vi "Create Transfer Configuration.vi"(7 "base transfer name (transfer)":string="transfer", 11 "channel count per transfer":i32) -> (3 "transfer configuration":T1)   [LabVIEW 2017]
uses:
  DSF.Shared.Refactor.Typedefs.Transfer Configuration.ctl
  DSF.Shared.Typedefs.Byte Order.ctl
  DSF.Shared.Refactor.Typedefs.Channel Array Configuration.ctl
  DSF.Shared.Typedefs.Data Type.ctl
  DSF.Shared.lvlib
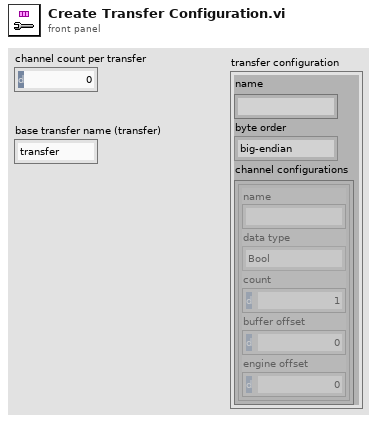
[diagram p1: front panel]
types:
  T1 = typedef "DSF.Shared.lvlib/DSF.Shared.Refactor.Typedefs.Transfer Configuration.ctl" = cluster{"name":string, "byte order":T2, "channel configurations":T3[]}
  T2 = typedef "DSF.Shared.lvlib/DSF.Shared.Typedefs.Byte Order.ctl" = enum8{"big-endian", "little-endian"}
  T3 = typedef "DSF.Shared.lvlib/DSF.Shared.Refactor.Typedefs.Channel Array Configuration.ctl" = cluster{"name":string, "data type":T4, "count":u64, "buffer offset":u64, "engine offset":u64}
  T4 = typedef "DSF.Shared.lvlib/DSF.Shared.Typedefs.Data Type.ctl" = enum8{"Bool", "SGL", "DBL", "I8", "I16", "I32", "I64", "U8", "U16", "U32", "U64"}
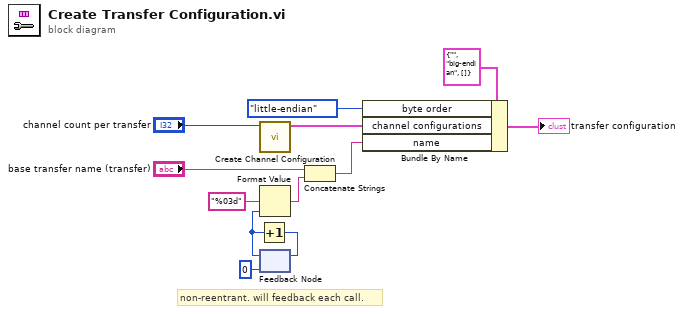
[diagram p0: block diagram]
diagram:
  # "non-reentrant. will feedback each call."
  n1 = call "Create Channel Configuration.vi"("channel count"="channel count per transfer") -> ("channel configurations"=w2:T3[])  [unwired: 9 in, 1 out]
  n2 = feedback #1(0) -> (w8:i32)
  n3 = Increment(x=w8) -> (x+1=w9:i32)
  n4 = Format Value(format string="%03d", value (0)=w8) -> (output string=w3:string)  [unwired: 1 in]
  n5 = feedback-in #1(w9) -> ()
  n6 = Concatenate Strings("base transfer name (transfer)", w3) -> (w1:string)
  n7 = Bundle By Name(cluster=T1 {"name"="", "byte order"=enum."big-endian", "channel configurations"=[]} ("Transfer Configuration"), "byte order"=DSF.Shared.Typedefs.Byte_Order."little-endian", "channel configurations"=w2, "name"=w1) -> (→"transfer configuration":T1)
